vi "Get Car Instance.vi"(7 "Car Name":string, 8 "error in (no error)":errorcluster, 11 "CarPool in":refnum<class "CarPool.lvclass">) -> (0 "error out":errorcluster, 1 "found":bool, 2 "Car":refnum<class "Car.lvclass">, 3 "CarPool out":refnum<class "CarPool.lvclass">)   [LabVIEW 2017, in "CarPool.lvclass"]
uses:
  CarPool.lvclass
  Car/Car.lvclass
  CarPool.lvclass/CarPool.ctl
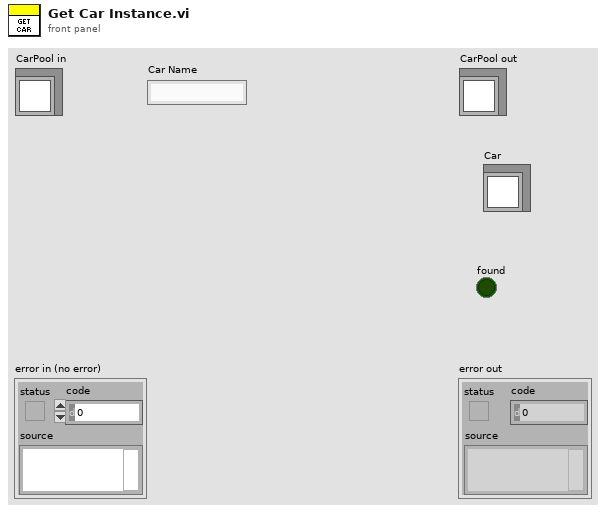
[diagram p1: front panel]
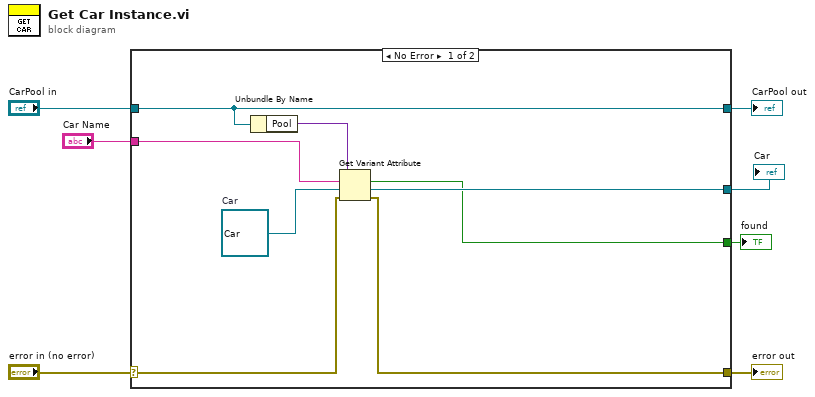
[diagram p0: block diagram]
diagram:
  n1 = case shown="No Error" "error in (no error)" {
    selector: "error in (no error)" -> [w9 w17]
    tunnel: [w8 w17] -> w6
    tunnel: [w11 w16] -> w4
    tunnel: "CarPool in" -> [w11 w16]
    tunnel: "Car Name" -> [w15 _]
    tunnel: [w13 _] -> w2
    tunnel: [w12 _] -> w1
    frame No Error {
      w14 = refnum<class "Car.lvclass"> refnum  # Car
      n2 = Unbundle By Name(w11) -> ("Pool"=w10:variant)
      n3 = Get Variant Attribute(Variant=w10, name=w15, default value (empty Variant)=w14, error in=w9) -> (found=w12:bool, value=w13:refnum<class "Car.lvclass">, error out=w8:errorcluster)  [unwired: 1 out]
    }
    frame Error {
    }
  }
  "error out" <- w6
  "CarPool out" <- w4
  "Car" <- w2
  "found" <- w1
